vi "Configure Chan Mode (Burst).vi"(4 "Width (10 msec)":dbl=0.01 format="%.6p", 6 "Delay (10 msec)":dbl=0.01 format="%.6p", 7 "Channel (1:Chan A)":i32(ring)=1 items=["Channel A"=1, "Channel B"=2, "Channel C"=3, "Channel D"=4, "Channel E"=5, "Channel F"=6, "Channel G"=7, "Channel H"=8], 8 "error in (no error)":errorcluster, 9 "Wait # (0)":i32, 10 "Burst # (10)":i32=10, 11 "VISA resource name":refnum<visa-resource-name>) -> (0 "error out":errorcluster, 3 "VISA resource name out":refnum<visa-resource-name>)   [LabVIEW 2019, in "Quantum Composers 9000 Series.lvlib"]
doc: "This VI is used to configure the burst mode of operation for a channel."
uses:
  Quantum Composers 9000 Series.lvlib
panel:
  # "Pulse Parameters"
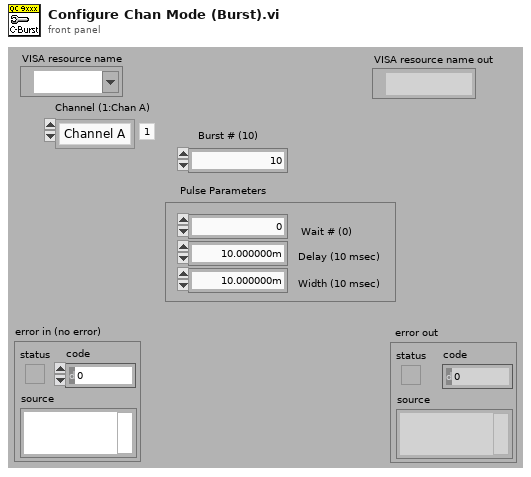
[diagram p1: front panel]
types:
  T1 = enum16{"Normal", "Single", "Burst", "Duty Cycle"}
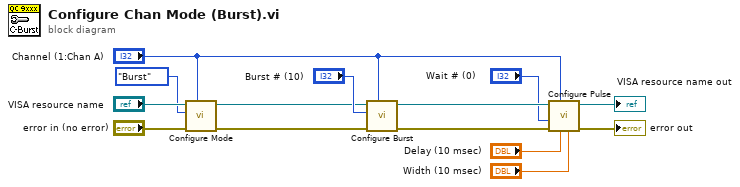
[diagram p0: block diagram]
diagram:
  n1 = call "Configure Mode.vi"("Channel (1:Chan A)"="Channel (1:Chan A)", "error in (no error)"="error in (no error)", "Mode (0:Normal)"=T1."Burst" ("Chan Mode"), "VISA resource name"="VISA resource name") -> ("error out"=w12:errorcluster, "VISA resource name out"=w13:refnum<visa-resource-name>)  [unwired: 6 in]
  n2 = call "Configure Burst.vi"("Channel (1:Chan A)"="Channel (1:Chan A)", "error in (no error)"=w12, "Burst # (10)"="Burst # (10)", "VISA resource name"=w13) -> ("error out"=w8:errorcluster, "VISA resource name out"=w7:refnum<visa-resource-name>)  [unwired: 6 in]
  n3 = call "Configure Pulse.vi"("Width (10 msec)"="Width (10 msec)", "Delay (10 msec)"="Delay (10 msec)", "Channel (1:Chan A)"="Channel (1:Chan A)", "error in (no error)"=w8, "Wait # (0)"="Wait # (0)", "VISA resource name"=w7) -> ("error out"=→"error out":errorcluster, "VISA resource name out"=→"VISA resource name out":refnum<visa-resource-name>)  [unwired: 4 in]
